vi "SynapseAPI-Change Mode.vi"(0 "URL":string="http://localhost:24414", 7 "mode":T1, 11 "error in (no error)":errorcluster) -> (15 "error out":errorcluster)   [LabVIEW 2020]
uses:
  SynapseAPI-Mode.ctl
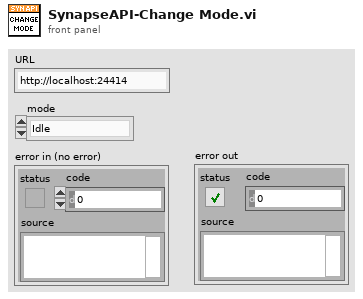
[diagram p1: front panel]
types:
  T1 = typedef "SynapseAPI-Mode.ctl" = enum16{"Idle", "Standby", "Preview", "Record"}
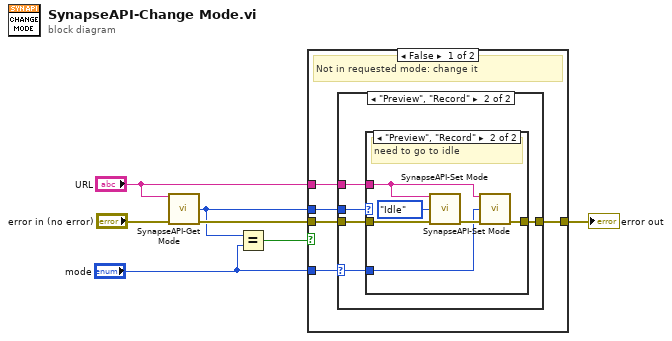
[diagram p0: block diagram]
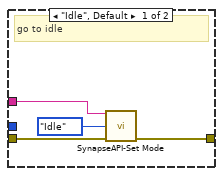
[diagram p2: hidden frame]
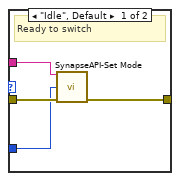
[diagram p3: hidden frame]
diagram:
  n1 = call "SynapseAPI-Get Mode.vi"("URL"="URL", "error in (no error)"="error in (no error)") -> ("mode"=w3:T1, "error out"=w5:errorcluster)  [unwired: 12 in]
  n2 = Equal?(x=w3, y="mode") -> (x = y?=w6:bool)
  n3 = case shown="False" w6 {
    tunnel: w5 -> [w9 w32]
    tunnel: "mode" -> [w12 _]
    tunnel: w3 -> [w11 _]
    tunnel: "URL" -> [w10 _]
    tunnel: [w8 w32] -> w1
    frame False {
      # "Not in requested mode: change it"
      n4 = case shown="\"Preview\", \"Record\"" w12 {
        selector: w12 -> [_ w18]
        tunnel: w11 -> [_ w21]
        tunnel: w10 -> [w14 w20]
        tunnel: w9 -> [w15 w19]
        tunnel: [w13 w17] -> w8
        frame "Idle", Default {
          # "go to idle"
          n5 = call "SynapseAPI-Set Mode.vi"("URL"=w14, "mode"=SynapseAPI-Mode."Idle", "error in (no error)"=w15) -> ("error out"=w13:errorcluster)  [unwired: 12 in]
        }
        frame "Preview", "Record" {
          n6 = case shown="\"Preview\", \"Record\"" w21 {
            tunnel: w20 -> [w25 w28]
            tunnel: w19 -> [w24 w31]
            tunnel: w18 -> [w23 w26]
            tunnel: [w22 w27] -> w17
            frame "Idle", Default {
              # "Ready to switch"
              n7 = call "SynapseAPI-Set Mode.vi"("URL"=w25, "mode"=w23, "error in (no error)"=w24) -> ("error out"=w22:errorcluster)  [unwired: 12 in]
            }
            frame "Preview", "Record" {
              # "need to go to idle"
              n8 = call "SynapseAPI-Set Mode.vi"("URL"=w28, "mode"=SynapseAPI-Mode."Idle", "error in (no error)"=w31) -> ("error out"=w29:errorcluster)  [unwired: 12 in]
              n9 = call "SynapseAPI-Set Mode.vi"("URL"=w28, "mode"=w26, "error in (no error)"=w29) -> ("error out"=w27:errorcluster)  [unwired: 12 in]
            }
          }
        }
      }
    }
    frame True {
      # "Already in requested mode"
    }
  }
  "error out" <- w1
